vi "Read Value.vi"(8 "error in (no error)":errorcluster, 11 "Waveform Array Result in":refnum<class "Waveform Array Result.lvclass">) -> (0 "error out":errorcluster, 2 "Value":dbl, 3 "Waveform Array Result out":refnum<class "Waveform Array Result.lvclass">)   [LabVIEW 2015, in "Waveform Array Result.lvclass"]
uses:
  Waveform Array Result.lvclass
  Waveform Array Result.lvclass/Waveform Array Result.ctl
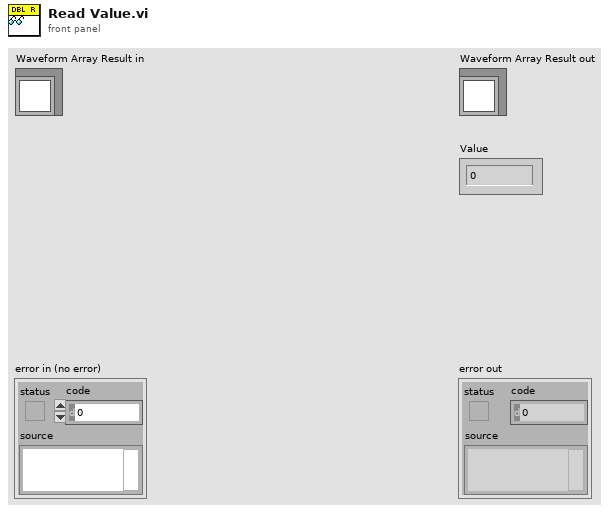
[diagram p1: front panel]
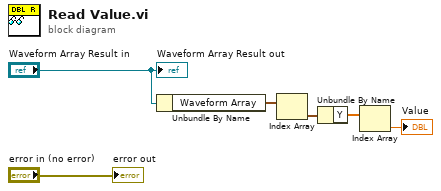
[diagram p0: block diagram]
diagram:
  n1 = Unbundle By Name("Waveform Array Result in") -> ("Waveform Array"=w6:waveform(dbl)[])
  n2 = Index Array(array=w6) -> (element=w5:waveform(dbl))  [unwired: 1 in]
  n3 = Unbundle By Name(w5) -> ("Y"=w4:dbl[])
  n4 = Index Array(array=w4) -> (element=→"Value":dbl)  [unwired: 1 in]
  "error out" <- "error in (no error)"
  "Waveform Array Result out" <- "Waveform Array Result in"
